vi "Validate N Factor.vi"(0 "N Factor":u8) -> (2 "N Factor":u8, 3 "Warning":string, 4 "Skip Number":dbl)   [LabVIEW 2019]
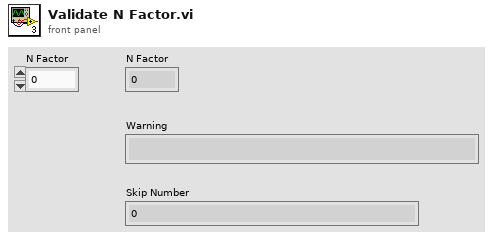
[diagram p1: front panel]
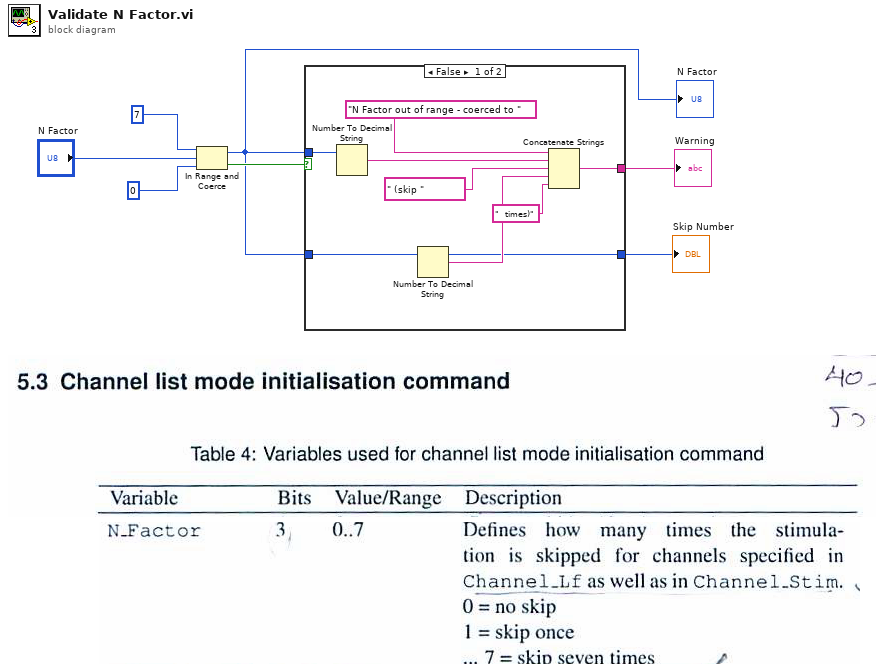
[diagram p0: block diagram]
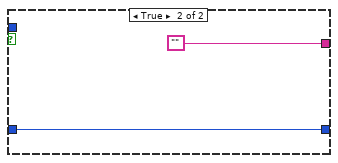
[diagram p2: hidden frame]
diagram:
  n1 = In Range and Coerce(upper limit=u16 7, x="N Factor", lower limit=i16 0) -> (coerced(x)=w1:u16, In Range?=w5:bool)
  "N Factor" <- w1
  n2 = case shown="False" w5 {
    tunnel: w1 -> [w12 _]
    tunnel: [w13 ""] -> w6
    tunnel: w1 -> [w8 w16]
    tunnel: [w8 w16] -> w7
    frame False {
      n3 = Number To Decimal String(number=w12) -> (decimal integer string=w14:string)  [unwired: 1 in]
      n4 = Number To Decimal String(number=w8) -> (decimal integer string=w10:string)  [unwired: 1 in]
      n5 = Concatenate Strings("N Factor out of range - coerced to ", w14, " (skip " ("string"), w10, "  times)" ("string")) -> (w13:string)
    }
    frame True {
    }
  }
  "Skip Number" <- w7
  "Warning" <- w6
